vi "Write Run Time Menu Properties.vi"(8 "error in (no error)":errorcluster, 10 "Run Time Menu Item":T1, 11 "RunTimeMenuItem in":refnum<class "RunTimeMenuItem.lvclass">) -> (0 "error out":errorcluster, 3 "RunTimeMenuItem out":refnum<class "RunTimeMenuItem.lvclass">)   [LabVIEW 2015, in "RunTimeMenuItem.lvclass"]
uses:
  RunTimeMenuItem.lvclass
  XML Controls/RunTimeMenus Properties.ctl
  XML Controls/Execution Types.ctl
  XML Controls/Path Cluster.ctl
  XML Controls/Dependency Properties.ctl
  RunTimeMenuItem.lvclass/RunTimeMenuItem.ctl
  VeriStand XML Parser.lvlib
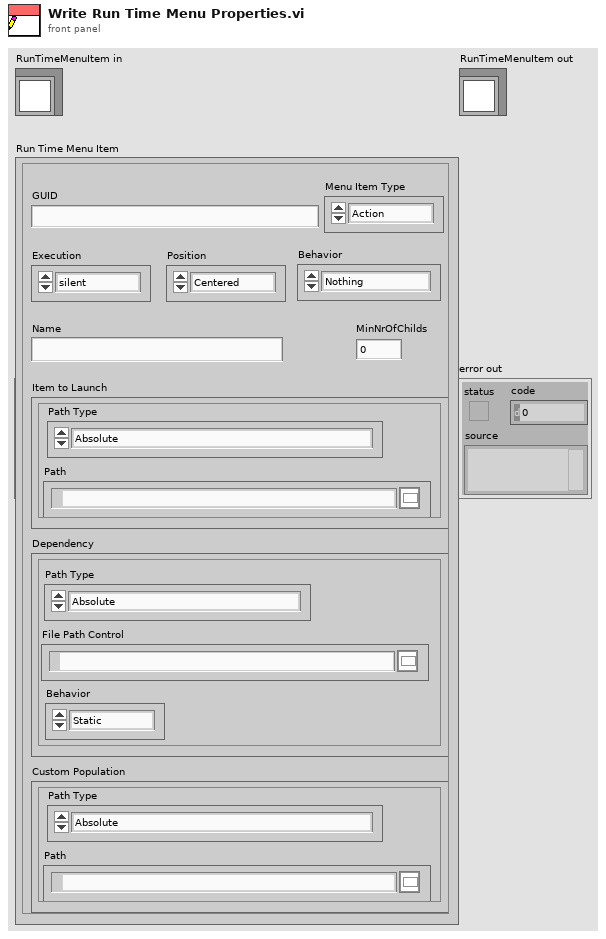
[diagram p1: front panel]
types:
  T1 = typedef "VeriStand XML Parser.lvlib/RunTimeMenus Properties.ctl" = cluster{"GUID":string, "Execution":T2, "MinNrOfChilds":u32, "Name":string, "Item to Launch":T3, "Dependency":T4, "Custom Population":T3, "Menu Item Type":enum16{"Action", "VI", "Separator", "Custom"}, "Behavior":enum16{"Nothing", "Open Front Panel"}, "Position":enum16{"Centered", "Mouse Pointer"}}
  T2 = typedef "VeriStand XML Parser.lvlib/Execution Types.ctl" = enum16{"silent", "modal", "floating", "default"}
  T3 = typedef "VeriStand XML Parser.lvlib/Path Cluster.ctl" = cluster{"Path":path, "Path Type":enum16{"Absolute", "To Base", "To Common Doc Dir", "To Application Data Dir"}}
  T4 = typedef "VeriStand XML Parser.lvlib/Dependency Properties.ctl" = cluster{"File Path Control":path, "Path Type":enum16{"Absolute", "To Base", "To Common Doc Dir", "To Application Data Dir"}, "Behavior":enum16{"Static", "Dynamic"}}
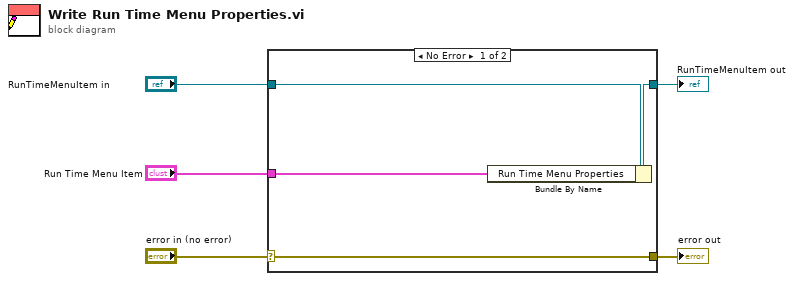
[diagram p0: block diagram]
diagram:
  n1 = case shown="No Error" "error in (no error)" {
    selector: "error in (no error)" -> [w9 w10]
    tunnel: [w9 w10] -> w4
    tunnel: [w7 w11] -> w2
    tunnel: "RunTimeMenuItem in" -> [w8 w11]
    tunnel: "Run Time Menu Item" -> [w6 _]
    frame No Error {
      n2 = Bundle By Name(cluster=w8, "Run Time Menu Properties"=w6) -> (w7:refnum<class "RunTimeMenuItem.lvclass">)
    }
    frame Error {
    }
  }
  "error out" <- w4
  "RunTimeMenuItem out" <- w2
